vi "Find API Tester Path.vi"(8 "error in":errorcluster, 11 "DQMH Library Ref":refnum<vi>) -> (0 "error out":errorcluster, 2 "Api tester found?":bool, 3 "API Tester Path":path)   [LabVIEW 2019, in "Panther Dashboard.lvlib"]
uses:
  Panther Dashboard.lvlib
  <vilib>/Utility/error.llb/Error Cluster From Error Code.vi
  Panther Dashboard--global.vi
  <vilib>/ErrorRing/Error Ring.xnode
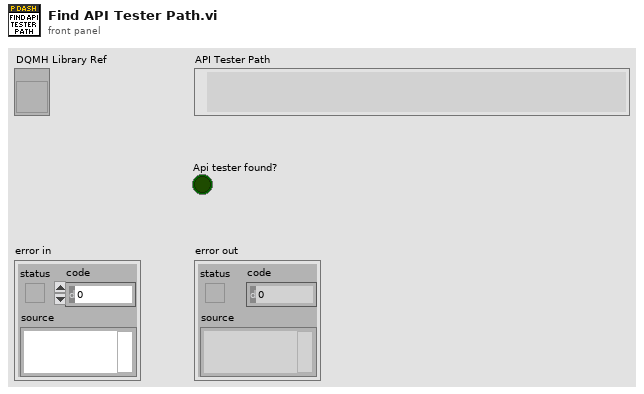
[diagram p1: front panel]
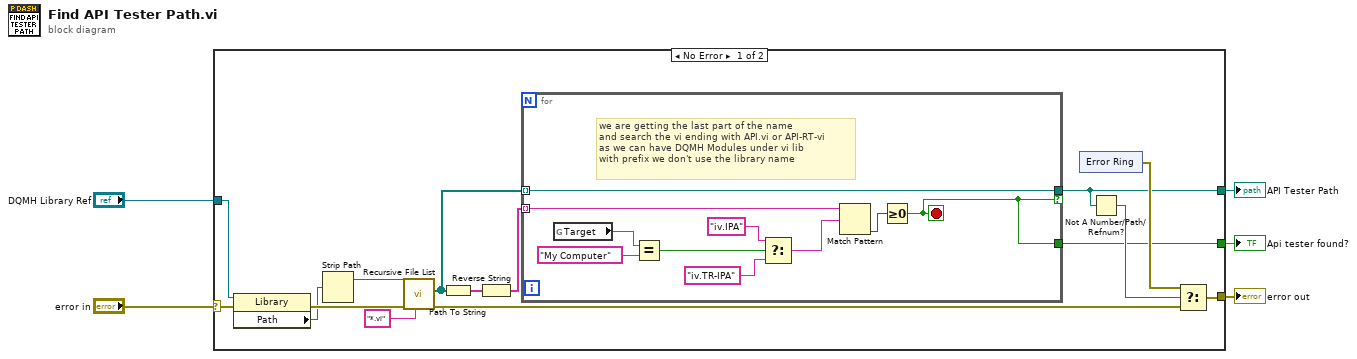
[diagram p0: block diagram]
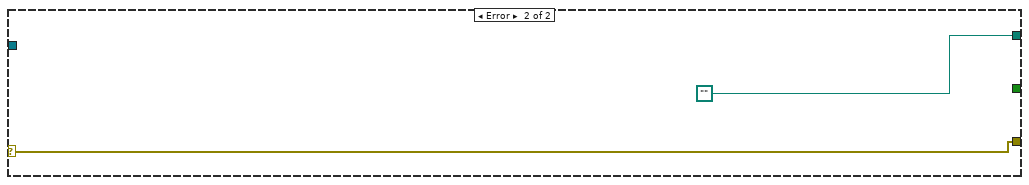
[diagram p2: hidden frame]
diagram:
  n1 = case shown="No Error" "error in" {
    selector: "error in" -> [w16 w37]
    tunnel: [w8 path ""] -> w3
    tunnel: [w18 w37] -> w4
    tunnel: "DQMH Library Ref" -> [w9 _]
    tunnel: [w6 _] -> w1
    frame No Error {
      n2 = property class="Library"(reference=w9, error in=w16) -> (error out=w17:errorcluster, "Path"=w10:path)  [unwired: 1 out]
      n3 = Strip Path(path=w10) -> (stripped path=w11:path)  [unwired: 1 out]
      n4 = call <vilib>:"Recursive File List.vi"("pattern"="*.vi", "error in (no error)"=w17, "Folder Path"=w11) -> ("error out"=w19:errorcluster, "All Files in Dir"=w12:path[])  [unwired: 4 in, 3 out]
      n5 = Path To String(path=w12) -> (string=w14:string[])
      n6 = Reverse String(1:w14) -> (0:w13:string[])
      n7 = for {
        tunnel: w13 -> [w34] mode=indexing
        tunnel: w12 -> [w35] mode=indexing
        tunnel: [w35] -> w8 if=w26
        tunnel: [w26] -> w6
        stop <- w26 stop-if-true
        # "we are getting the last part of the name\nand search the vi ending with API.vi or API-RT-vi\nas we can have DQMH Modules under vi lib\nwith prefix we don't use the library name"
        n8 = global read "Panther Dashboard--global.vi" "Target"() -> (w32:string)
        n9 = Equal?(x=w32, y="My Computer") -> (x = y?=w30:bool)
        n10 = Select(t="iv.IPA", s=w30, f="iv.TR-IPA") -> (s? t:f=w28:string)
        n11 = Match Pattern(string=w34, regular expression=w28) -> (offset past match=w33:i32)  [unwired: 1 in, 3 out]
        n12 = Greater Or Equal To 0?(x=w33) -> (x >= 0?=w26:bool)
      }
      n13 = xnode "Error Ring"() -> ("error out"=w20:errorcluster)
      n14 = Not A Number/Path/Refnum?(number/path/refnum=w8) -> (NaN/Path/Refnum?=w7:bool)
      n15 = Select(t=w20, s=w7, f=w19) -> (s? t:f=w18:errorcluster)
    }
    frame Error {
    }
  }
  "API Tester Path" <- w3
  "error out" <- w4
  "Api tester found?" <- w1
